vi "Click Position.vi"(8 "error in (no error)":errorcluster, 9 "Timeline Ref":T3, 11 "Click Coords":T2) -> (0 "error out":errorcluster, 3 "Operation":T1)   [LabVIEW 2013, in "XGrapher.xctl"]
doc: "Determines the area in which the operator is mousing in. This will determine the mouse cursor to use"
uses:
  XGrapher.xctl
  Typedefs/Xctrl-Timeline graph ref.ctl
  <vilib>/Utility/miscctls.llb/LVPoint32TypeDef.ctl
  Typedefs/Xcrtl-Click Operation.ctl
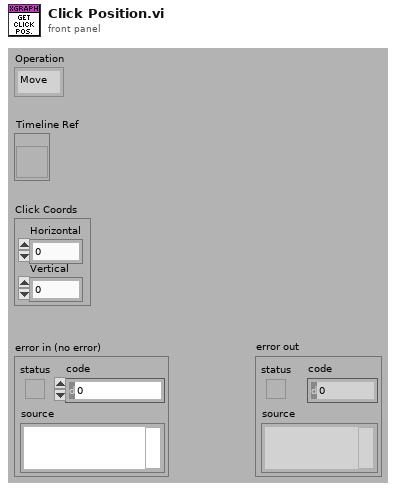
[diagram p1: front panel]
types:
  T1 = typedef "XGrapher.xctl/Xcrtl-Click Operation.ctl" = enum16{"Move", "left cursor", "right cursor", "none"}
  T2 = typedef "LVPoint32TypeDef.ctl" = cluster{"Horizontal":i32, "Vertical":i32}
  T3 = typedef "XGrapher.xctl/Xctrl-Timeline graph ref.ctl" = refnum<vi>
  T4 = cluster{"Left cursor pos.":dbl, "Left cursor pos.":dbl}
  T5 = cluster{"Right cursor pos.":dbl, "Right cursor pos.":dbl}
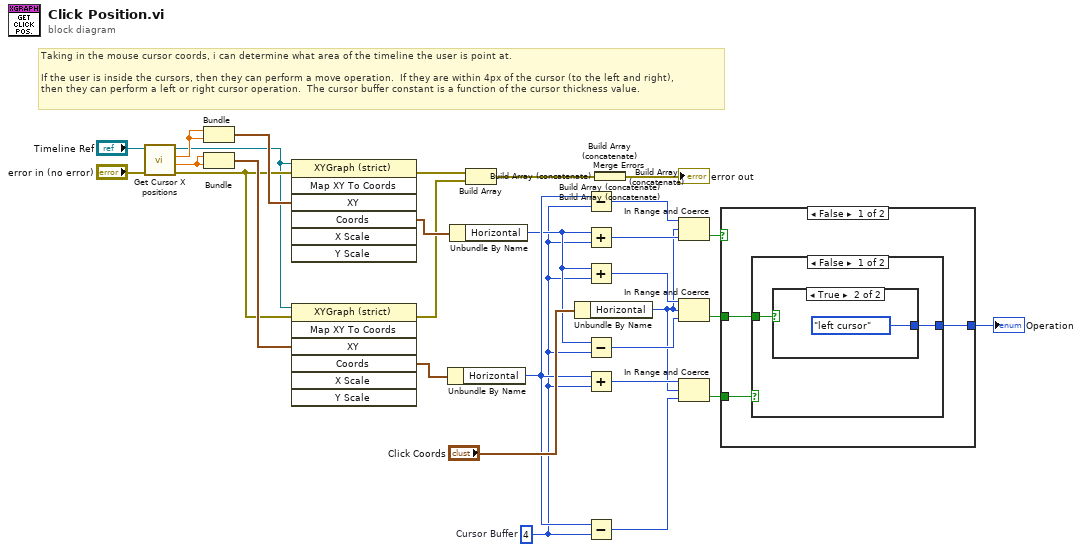
[diagram p0: block diagram]
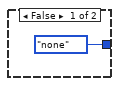
[diagram p2: hidden frame]
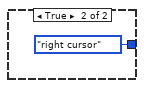
[diagram p3: hidden frame]
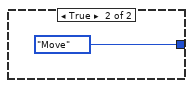
[diagram p4: hidden frame]
diagram:
  w18 = 4  # Cursor Buffer
  # "Taking in the mouse cursor coords, i can determine what area of the timeline the user is point at.\n\nIf the user is inside the cursors, then they can perform a move operation.  If they are within 4px of the cursor (to the left and right),\nthen they can perform a left or right cursor operation.  The cursor buffer constant is a function of the cursor thickness value."
  n1 = call "Get Cursor X positions.vi"("error in"="error in (no error)", "Timeline Graph"="Timeline Ref") -> ("error out"=w14:errorcluster, "Right cursor pos."=w4:dbl, "Left cursor pos."=w3:dbl, "Timeline Graph out"=w1:T3)  [unwired: 5 in, 1 out]
  n2 = Bundle("Left cursor pos."=w3, "Left cursor pos."=w3) -> (w30:T4)  [unwired: 1 in]
  n3 = Bundle("Right cursor pos."=w4, "Right cursor pos."=w4) -> (w34:T5)  [unwired: 1 in]
  n4 = invoke on="Invoke Node" class="XYGraph (strict)" method="Map XY To Coords"(reference=w1, error in=w14, "XY"=w30) -> (error out=w13:errorcluster, "Coords"=w31:T2)  [unwired: 4 in, 5 out]
  n5 = invoke on="Invoke Node" class="XYGraph (strict)" method="Map XY To Coords"(reference=w1, error in=w14, "XY"=w34) -> (error out=w12:errorcluster, "Coords"=w33:T2)  [unwired: 4 in, 5 out]
  n6 = Unbundle By Name(w33) -> ("Horizontal"=w25:i32)
  n7 = Unbundle By Name(w31) -> ("Horizontal"=w19:i32)
  n8 = Build Array(w13, w12) -> (w10:errorcluster[])
  n9 = Unbundle By Name("Click Coords") -> ("Horizontal"=w17:i32)
  n10 = Subtract(x=w25, y=w18) -> (x-y=w28:i32)
  n11 = Add(x=w19, y=w18) -> (x+y=w29:i32)
  n12 = Add(x=w19, y=w18) -> (x+y=w20:i32)
  n13 = Subtract(x=w19, y=w18) -> (x-y=w21:i32)
  n14 = Add(x=w25, y=w18) -> (x+y=w24:i32)
  n15 = Subtract(x=w25, y=w18) -> (x-y=w23:i32)
  n16 = Build Array (concatenate)(w10) -> (w9:errorcluster[])
  n17 = Build Array (concatenate)(w9) -> (w8:errorcluster[])
  n18 = Build Array (concatenate)(w8) -> (w7:errorcluster[])
  n19 = Build Array (concatenate)(w7) -> (w6:errorcluster[])
  n20 = Build Array (concatenate)(w6) -> (w5:errorcluster[])
  n21 = Merge Errors(w5) -> (→"error out":errorcluster)
  n22 = In Range and Coerce(upper limit=w28, x=w17, lower limit=w29) -> (In Range?=w27:bool)  [unwired: 1 out]
  n23 = In Range and Coerce(upper limit=w20, x=w17, lower limit=w21) -> (In Range?=w16:bool)  [unwired: 1 out]
  n24 = In Range and Coerce(upper limit=w24, x=w17, lower limit=w23) -> (In Range?=w22:bool)  [unwired: 1 out]
  n25 = case shown="False" w27 {
    tunnel: [w37 Xcrtl-Click_Operation."Move" ("Operation")] -> w26
    tunnel: w22 -> [w36 _]
    tunnel: w16 -> [w35 _]
    frame False {
      n26 = case shown="False" w36 {
        tunnel: [w39 Xcrtl-Click_Operation."right cursor" ("Operation")] -> w37
        tunnel: w35 -> [w38 _]
        frame False {
          n27 = case shown="True" w38 {
            tunnel: [Xcrtl-Click_Operation."none" ("Operation") Xcrtl-Click_Operation."left cursor" ("Operation")] -> w39
            frame False {
            }
            frame True {
            }
          }
        }
        frame True {
        }
      }
    }
    frame True {
    }
  }
  "Operation" <- w26
